vi "Close.vi"(8 "error in (no error)":errorcluster, 11 "Abstract_Mono in":refnum<class "Abstract_Mono.lvclass">) -> (0 "error out":errorcluster, 3 "Abstract_Mono out":refnum<class "Abstract_Mono.lvclass">)   [LabVIEW 2020, in "Abstract_Mono.lvclass"]
uses:
  <instrlib>/Classes/Monochromator/Monochromator_Abstract/Abstract_Mono.lvclass
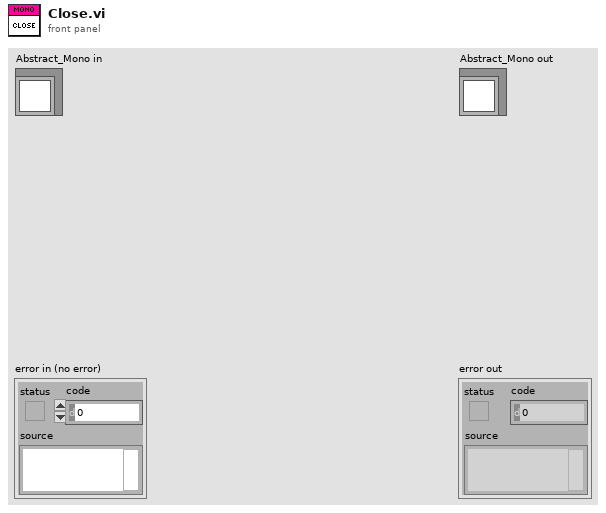
[diagram p1: front panel]
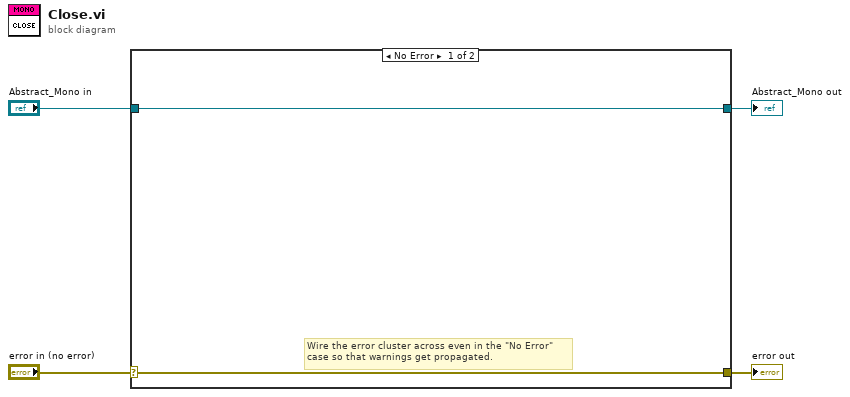
[diagram p0: block diagram]
diagram:
  n1 = case shown="No Error" "error in (no error)" {
    selector: "error in (no error)" -> [w5 w8]
    tunnel: [w5 w8] -> w3
    tunnel: [w6 w7] -> w1
    tunnel: "Abstract_Mono in" -> [w6 w7]
    frame No Error {
      # "Wire the error cluster across even in the \"No Error\"\ncase so that warnings get propagated."
    }
    frame Error {
    }
  }
  "error out" <- w3
  "Abstract_Mono out" <- w1
